vi "test5-Broadcast_Queue.vi"(8 "error in (no error)":errorcluster, 11 "TestCase in":refnum<class "testcase-CSMGlobalLog.lvclass">) -> (0 "error out":errorcluster, 3 "TestCase out":refnum<class "testcase-CSMGlobalLog.lvclass">)   [LabVIEW 2017, in "testcase-CSMGlobalLog.lvclass"]
uses:
  testcase-CSMGlobalLog.lvclass
  testcase-CSMGlobalLog.lvclass/testcase-CSMGlobalLog.ctl
  ff5deddd-bde5-43e0-b60c-bddac20d3018.vi
  <vilib>/addons/_JKI Toolkits/VI Tester/TestCase.llb/TestCase.lvclass
  src/user.lib/_NEVSTOP/Communicable State Machine(CSM)/Utility/Periodic String Filter Setting.ctl
  src/user.lib/_NEVSTOP/Communicable State Machine(CSM)/Communicable State Machine.lvlib
  CSM/CSM-Testcase.lvlib
  C:/Program Files (x86)/National Instruments/LabVIEW 2017/vi.lib/addons/_JKI Toolkits/VI Tester/TestCase.llb/TestCase.lvclass
panel:
  out "String cache total":string
  out "LoopCount":i32
  out "String Cache Each Loop":string
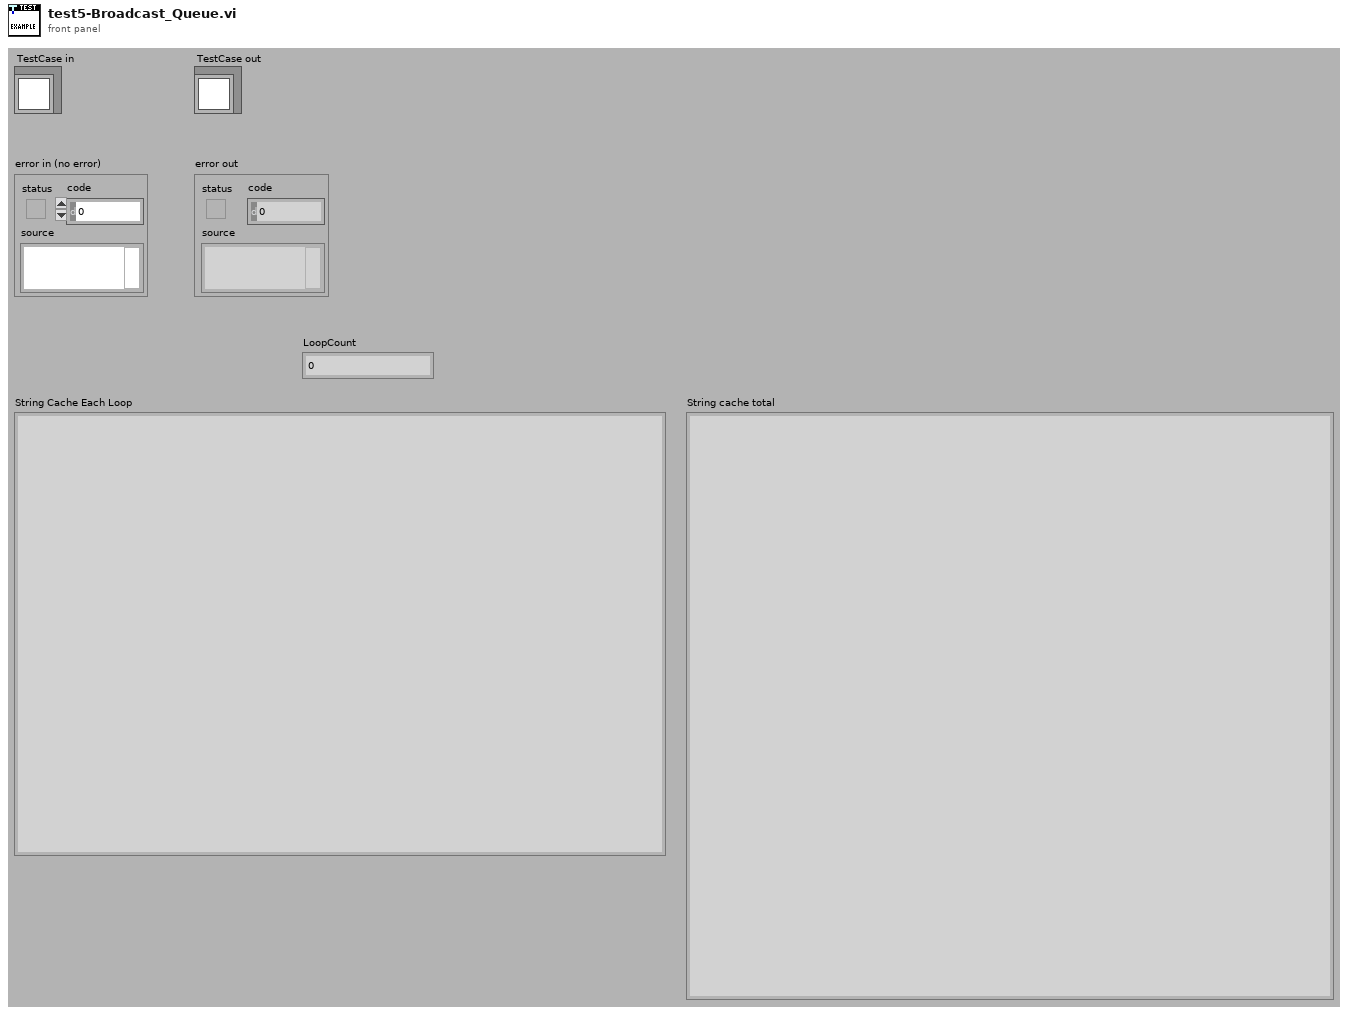
[diagram p1: front panel]
types:
  T1 = typedef "Communicable State Machine.lvlib/Periodic String Filter Setting.ctl" = cluster{"threashold(#/s)":dbl, "Check Peroid(s)":dbl}
  T2 = typedef "Communicable State Machine.lvlib/_CSM_GlobalLog_MSG.ctl" = cluster{"Name (\"\" to Use UUID)":string, "Current State":string, "Arguments":string, "Source Message":T3, "Source Module":string, "Complete(T)/Start(F)":bool, "LogType":T4, "Time Stamp":timestamp}
  T3 = typedef "Communicable State Machine.lvlib/_CSM_Response Source Message.ctl" = cluster{"‘State":string, "’Arguments":string, "’Error":errorcluster}
  T4 = typedef "Communicable State Machine.lvlib/_CSM_GlobalLog_MSG_TYPE.ctl" = enum16{"User Log", "State Change", "Status", "Interrupt", "Register", "Unregister", "Error Log", "Module Created", "Module Destroyed", "Async Message", "No-Rep Async Message", "Sync Message"}
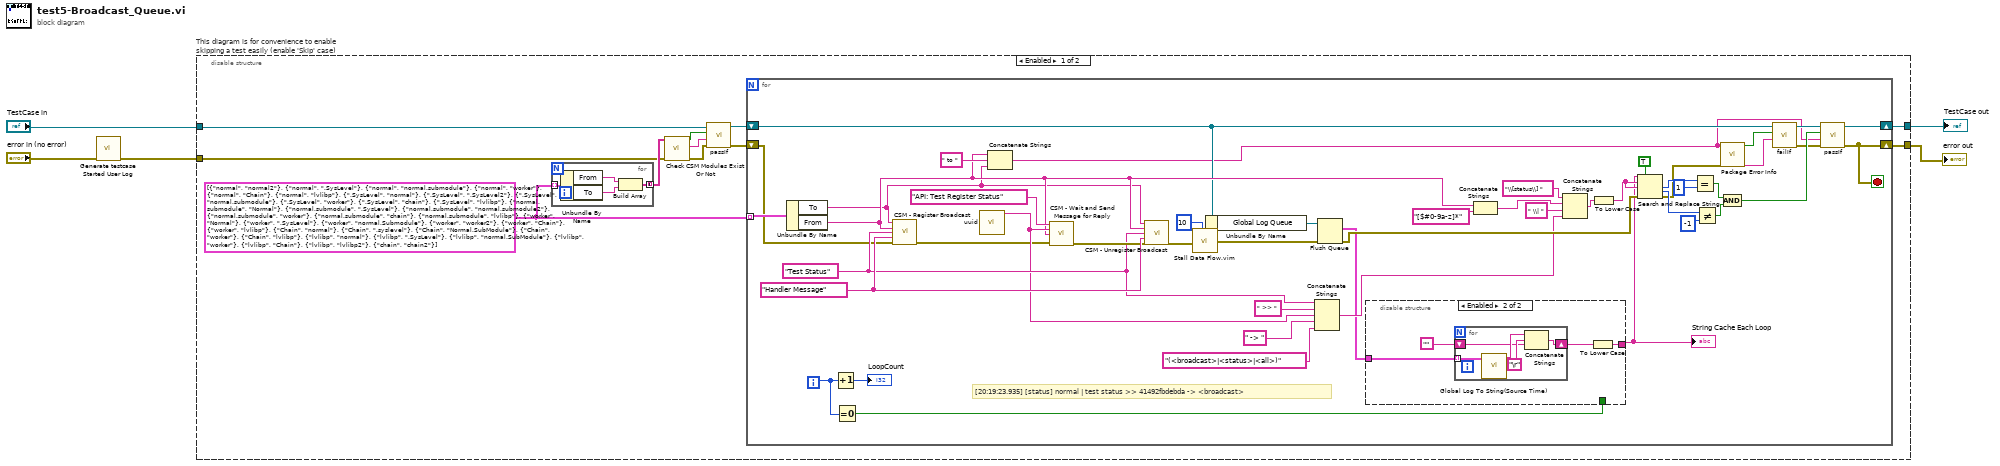
[diagram p0: block diagram]
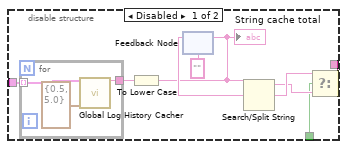
[diagram p2: hidden frame]
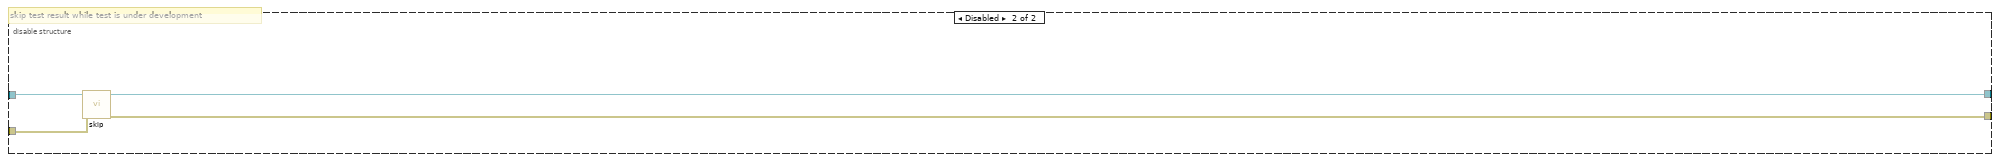
[diagram p3: hidden frame]
diagram:
  n1 = call "Generate testcase Started User Log.vi"("Error In"="error in (no error)") -> ("error out"=w1:errorcluster)  [unwired: 10 in]
  n2 = disable-structure "This diagram is for convenience to enable skipping a test easily (enable 'Skip' case)" shown="Enabled" {
    disable-tunnel: "TestCase in" -> [w9 w93]
    disable-tunnel: [w15 w91] -> w2
    disable-tunnel: [w16 w92] -> w4
    disable-tunnel: w1 -> [w6 w90]
    frame Enabled {
      w10 = cluster{"From":string, "To":string}[] [{"From"="normal", "To"="normal2"}, {"From"="normal", "To"=".SysLevel"}, {"From"="normal", "To"="normal.submodule"}, {"From"="normal", "To"="worker"}, {"From"="normal", "To"="Chain"}, {"From"="normal", "To"="lvlibp"}, {"From"=".SysLevel", "To"="normal"}, {"From"=".SysLevel", "To"=".SysLevel2"}, {"From"=".SysLevel", "To"="normal.submodule"}, {"From"=".SysLevel", "To"="worker"}, {"From"=".SysLevel", "To"="chain"}, {"From"=".SysLevel", "To"="lvlibp"}, {"From"="normal.submodule", "To"="Normal"}, {"From"="normal.submodule", "To"=".SysLevel"}, {"From"="normal.submodule", "To"="normal.submodule2"}, {"From"="normal.submodule", "To"="worker"}, {"From"="normal.submodule", "To"="chain"}, {"From"="normal.submodule", "To"="lvlibp"}, {"From"="worker", "To"="Normal"}, {"From"="worker", "To"=".SysLevel"}, {"From"="worker", "To"="normal.Submodule"}, {"From"="worker", "To"="worker2"}, {"From"="worker", "To"="Chain"}, {"From"="worker", "To"="lvlibp"}, {"From"="Chain", "To"="normal"}, {"From"="Chain", "To"=".syslevel"}, {"From"="Chain", "To"="Normal.SubModule"}, {"From"="Chain", "To"="worker"}, {"From"="Chain", "To"="lvlibp"}, {"From"="lvlibp", "To"="normal"}, {"From"="lvlibp", "To"=".SysLevel"}, {"From"="lvlibp", "To"="normal.SubModule"}, {"From"="lvlibp", "To"="worker"}, {"From"="lvlibp", "To"="Chain"}, {"From"="lvlibp", "To"="lvlibp2"}, {"From"="chain", "To"="chain2"}]
      n3 = for {
        tunnel: w10 -> [w20] mode=indexing
        tunnel: [w17] -> w13 mode=concatenating
        n4 = Unbundle By Name(w20) -> ("From"=w19:string, "To"=w18:string)
        n5 = Build Array(w19, w18) -> (w17:string[])
      }
      n6 = call "Check CSM Modules Exist Or Not.vi"("error in"=w6, "CSM names in"=w13) -> ("error out"=w11:errorcluster, "Debug string"=w12:string, "All Modules Exist?"=w14:bool)  [unwired: 7 in]
      n7 = call-dynamic "passIf.vi"("error in (no error)"=w11, "message (\"\")"=w12, "pass"=w14, "TestCase in"=w9) -> ("error out"=w7:errorcluster, "TestCase out"=w8:refnum<class "testcase-CSMGlobalLog.lvclass">)  [unwired: 6 in]
      n8 = for {
        tunnel: w10 -> [w56] mode=indexing
        shift-right: [w39] -> w16
        shift-left: w7 -> [w31]
        shift-right: [w68] -> w15
        shift-left: w8 -> [w25]
        i -> [w33]
        stop <- w39 stop-if-true
        w55 = "Handler Message" ("API (If \"\", Same as Trigger)")
        w48 = "Test Status" ("Trigger")
        # "[20:19:23.935] [status] normal | test status >> 41492fbdebda -> <broadcast>"
        n9 = Unbundle By Name(w56) -> ("To"=w28:string, "From"=w29:string)
        n10 = Increment(x=w33) -> (x+1=→"LoopCount":i32)
        n11 = Equal To 0?(x=w33) -> (x = 0?=w32:bool)
        n12 = call "CSM - Register Broadcast.vi"("CSM Name(Empty for Broadcast Event)"=w28, "Source CSM Name (* as Default)"=w29, "Trigger"=w48, "API (If \"\", Same as Trigger)"=w55, "Error In"=w31) -> ("error out"=w40:errorcluster)  [unwired: 9 in, 1 out]
        n13 = call "uuid.vi"() -> ("UUID"=w46:string)  [unwired: 11 in]
        n14 = Concatenate Strings(w29, " to " ("string"), w28) -> (w21:string)
        n15 = call "CSM - Wait and Send Message for Reply.vi"("State"="API: Test Register Status", "Arguments (\"\")"=w46, "Target Module"=w29, "Error In (No Error)"=w40) -> ("error out"=w53:errorcluster)  [unwired: 8 in, 3 out]
        n16 = call "CSM - Unregister Broadcast.vi"("CSM Name(Empty for Broadcast Event)"=w28, "Source CSM Name (* as Default)"=w29, "Trigger"=w48, "API (\"*\" as Default)"=w55, "Error In"=w53) -> ("error out"=w38:errorcluster)  [unwired: 9 in, 1 out]
        n17 = call "Stall Data Flow.vim"("value in"=w38, "milliseconds to wait"=u32 10) -> ("value out"=w37:errorcluster)  [unwired: 1 out]
        n18 = Unbundle By Name(w25) -> ("Global Log Queue"=w67:refnum<queue>)
        n19 = Concatenate Strings(w48, " >> " ("string"), w46, " -> " ("string"), "(<broadcast>|<status>|<all>)" ("search string")) -> (w44:string)
        n20 = Flush Queue(queue=w67, error in (no error)=w37) -> (remaining elements=w35:T2[], error out=w58:errorcluster)  [unwired: 1 out]
        n21 = disable-structure shown="Enabled" {
          disable-tunnel: [w71 w81] -> w34
          disable-tunnel: w32 -> [w70 _]
          disable-tunnel: w35 -> [w69 w83]
          frame Disabled {
            n22 = for {
              tunnel: w69 -> [w80] mode=indexing
              tunnel: [w79] -> w77
              n23 = call "Global Log History Cacher.vi"("Global Log Data"=w80, "Settings"=T1 {"threashold(#/s)"=0.5, "Check Peroid(s)"=5.0}) -> ("String Cache"=w79:string)  [unwired: 13 in]
            }
            n24 = To Lower Case(string=w77) -> (all lower case string=w72:string)
            "String cache total" <- w72
            n25 = feedback #1("") -> (w76:string)
            n26 = feedback-in #1(w72) -> ()
            n27 = Search/Split String(string=w72, search string/char (-)=w76) -> (substring before match=w73:string, match + rest of string=w74:string)  [unwired: 1 in, 1 out]
            n28 = Select(t=w74, s=w70, f=w73) -> (s? t:f=w71:string)
          }
          frame Enabled {
            n29 = for {
              tunnel: w83 -> [w89] mode=indexing
              shift-right: [w85] -> w82
              shift-left: "" -> [w86]
              n30 = call "Global Log To String(Source Time).vi"("Log"=w89) -> ("Log String"=w88:string)  [unwired: 9 in]
              n31 = Concatenate Strings(w88, "\r", w86) -> (w85:string)
            }
            n32 = To Lower Case(string=w82) -> (all lower case string=w81:string)
          }
        }
        "String Cache Each Loop" <- w34
        n33 = Concatenate Strings(w29, "[$#0-9a-z]*" ("string")) -> (w41:string)
        n34 = Concatenate Strings("\\[status\\] " ("regular expression"), w41, " \\| " ("string"), w44) -> (w51:string)
        n35 = To Lower Case(string=w51) -> (all lower case string=w64:string)
        n36 = Search and Replace String(replace all?=TRUE ("replace all? (F)"), input string=w34, search string=w64, replace string=w64, error in=w58) -> (number of replacements=w63:i32, offset past replacement=w62:i32, error out=w22:errorcluster)  [unwired: 3 in, 1 out]
        n37 = Equal?(x=w63, y=1) -> (x = y?=w60:bool)
        n38 = Not Equal?(x=w62, y=-1) -> (x != y?=w59:bool)
        n39 = call "Package Error Info.vi"("error in"=w22, "String in"=w21) -> ("packed error info out"=w26:string, "error status"=w27:bool)  [unwired: 8 in]
        n40 = And(x=w60, y=w59) -> (x .and. y?=w49:bool)
        n41 = call-dynamic "failIf.vi"("message (\"\")"=w26, "fail"=w27, "TestCase in"=w25) -> ("error out"=w23:errorcluster, "TestCase out"=w24:refnum<class "testcase-CSMGlobalLog.lvclass">)  [unwired: 7 in]
        n42 = call-dynamic "passIf.vi"("error in (no error)"=w23, "message (\"\")"=w21, "pass"=w49, "TestCase in"=w24) -> ("error out"=w39:errorcluster, "TestCase out"=w68:refnum<class "testcase-CSMGlobalLog.lvclass">)  [unwired: 6 in]
      }
    }
    frame Disabled {
      # "skip test result while test is under development"
      n43 = call <vilib>:"skip.vi"("error in (no error)"=w90, "TestCase in"=w93) -> ("error out"=w92:errorcluster, "TestCase out"=w91:refnum<class "testcase-CSMGlobalLog.lvclass">)  [unwired: 8 in]
    }
  }
  "error out" <- w4
  "TestCase out" <- w2
